vi "I32 TO hex.vi"(11 "x":i32=32700327) -> (3 "concatenated string":string)   [LabVIEW 2017]
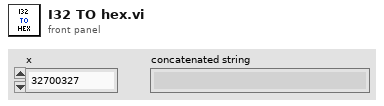
[diagram p1: front panel]
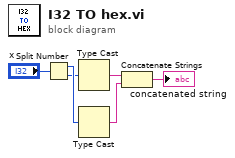
[diagram p0: block diagram]
diagram:
  n1 = Split Number(x="x") -> (hi(x)=w4:u16, lo(x)=w3:u16)
  n2 = Type Cast(x=w3) -> (*(type *) &x=w2:string)  [unwired: 1 in]
  n3 = Type Cast(x=w4) -> (*(type *) &x=w1:string)  [unwired: 1 in]
  n4 = Concatenate Strings(w2, w1) -> (→"concatenated string":string)
